vi "requestJobNameList.vi"(8 "error in (no error)":errorcluster, 10 "Storage location":u16(ring)=1 items=["Flash"=1, "USB"=2], 11 "SM1000-control in":T1) -> (0 "error out":errorcluster, 1 "Job name list":string, 2 "Job count":i32, 3 "SM1000-control out":T1)   [LabVIEW 2013, in "MaterialCharacterization.lvlib" / "MC-SM1000.lvclass"]
doc: "Gets a list of job names stored on the EC1000 Flash or USB Flash.\n\nReturns a list of jobs stored in the specified storage location on the EC1000."
uses:
  MC-SM1000.lvclass
  Object-reference.ctl
  MC-SM1000.lvclass/MC-SM1000.ctl
  Custom-errors.ctl
  C:/Users/vangeste/Desktop/2015-06-02 - SLM - MAIF/HC-HardwareCharacterization/Sources/SM1000/LECSession.dll
  HC-HardwareCharacterization/Sources/SM1000/LECSession.dll
  DOTNET-error-int.vi
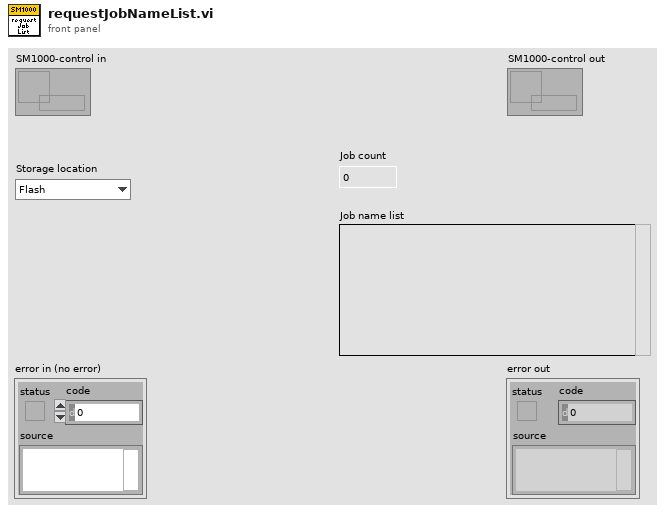
[diagram p1: front panel]
types:
  T1 = typedef "MaterialCharacterization.lvlib/MC-SM1000.lvclass/Object-reference.ctl" = refnum<data-value>
  T2 = typedef "MaterialCharacterization.lvlib/MC-SM1000.lvclass/Custom-errors.ctl" = enum16{"No error", "Not implemented", "Command not recognized", "Invalid input", "No connection", "Timeout", "Resource not loaded"}
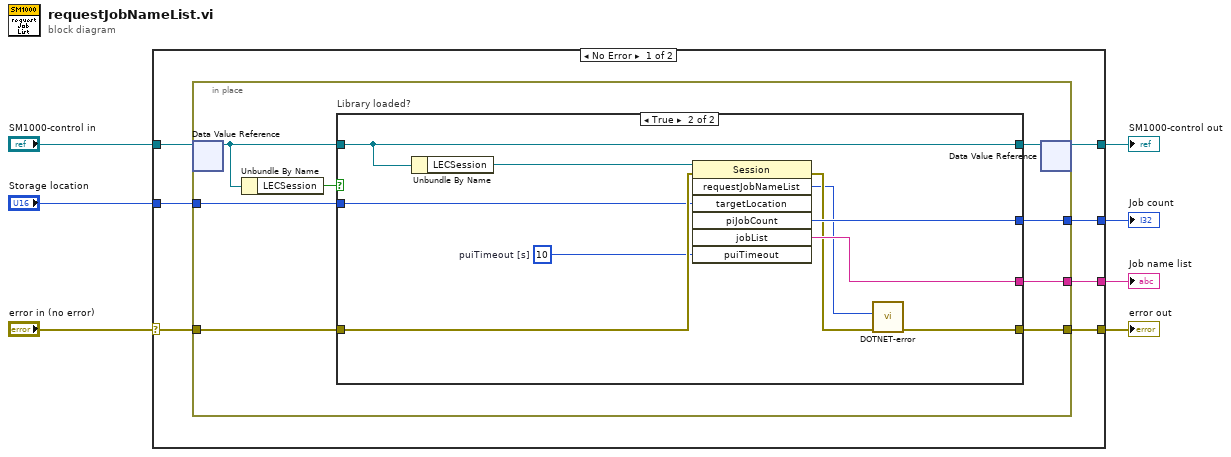
[diagram p0: block diagram]
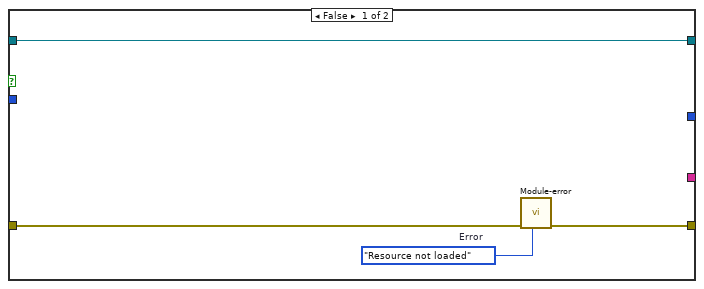
[diagram p2: hidden frame]
diagram:
  n1 = case shown="No Error" "error in (no error)" {
    selector: "error in (no error)" -> [w12 w38]
    tunnel: [w11 w38] -> w6
    tunnel: [w13 w37] -> w4
    tunnel: "SM1000-control in" -> [w14 w37]
    tunnel: "Storage location" -> [w10 _]
    tunnel: [w9 _] -> w2
    tunnel: [w8 _] -> w1
    frame No Error {
      n2 = in-place {
        in-place-border: w12 -> [w22]
        in-place-border: [w19] -> w11
        in-place-border: w10 -> [w17]
        in-place-border: [w16] -> w9
        in-place-border: [w15] -> w8
        n3 = in-place-dvr #1(w14) -> (w20:refnum<class "MC-SM1000.lvclass">)  [unwired: 1 out]
        n4 = Unbundle By Name(w20) -> ("LECSession"=w21:bool)
        n5 = case "Library loaded?" shown="True" w21 {
          tunnel: w22 -> [w26 w35]
          tunnel: w20 -> [w24 w34]
          tunnel: [w25 w29] -> w19
          tunnel: [w24 w34] -> w18
          tunnel: w17 -> [_ w33]
          tunnel: [_ w32] -> w16
          tunnel: [_ w31] -> w15
          frame False {
            w23 = Custom-errors."Resource not loaded"  # Error
            n6 = call "Module-error.vi"("Error"=w23, "error in (no error)"=w26) -> ("error out"=w25:errorcluster)  [unwired: 9 in]
          }
          frame True {
            w30 = u32 10  # puiTimeout [s]
            n7 = Unbundle By Name(w34) -> ("LECSession"=w36:refnum<k24>)
            n8 = invoke class="Session" method="requestJobNameList"(reference=w36, error in=w35, "targetLocation"=w33, "puiTimeout"=w30) -> (error out=w28:errorcluster, "requestJobNameList"=w27:u32, "piJobCount"=w32:i32, "jobList"=w31:string)  [unwired: 3 in, 3 out]
            n9 = call-poly "DOTNET-error.vi"("error in (no error)"=w28, "Retun code"=w27) -> ("error out"=w29:errorcluster)  [unwired: 9 in]
          }
        }
        n10 = in-place-dvr #1(w18) -> (w13:T1)  [unwired: 1 out]
      }
    }
    frame Error {
    }
  }
  "error out" <- w6
  "SM1000-control out" <- w4
  "Job name list" <- w1
  "Job count" <- w2
